vi "file paths.vi"(6 "error in (no error)":errorcluster, 7 "file path control":T1) -> (1 "ini":T2, 2 "coaglog":refnum<k34>, 4 "error out":errorcluster, 5 "datalog":refnum<k34>)   [LabVIEW 2019]
uses:
  <vilib>/Utility/config.llb/Config Data RefNum.ctl
  file paths.ctl
  <vilib>/Utility/config.llb/NI_LVConfig.lvlib
panel:
  out "appended path":path
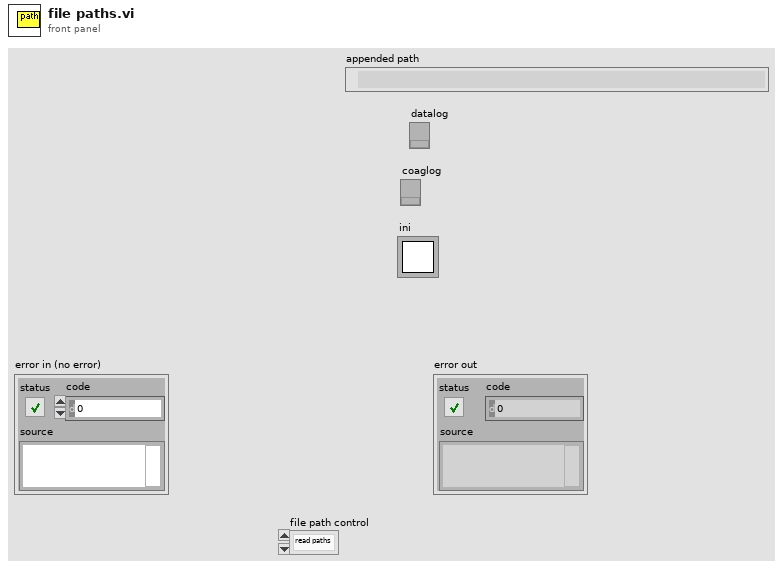
[diagram p1: front panel]
types:
  T1 = typedef "file paths.ctl" = enum16{"read paths", "close"}
  T2 = typedef "NI_LVConfig.lvlib/Config Data RefNum.ctl" = refnum<k1>
  T3 = enum16{"open", "open or create", "create or replace", "create", "open (read-only)"}
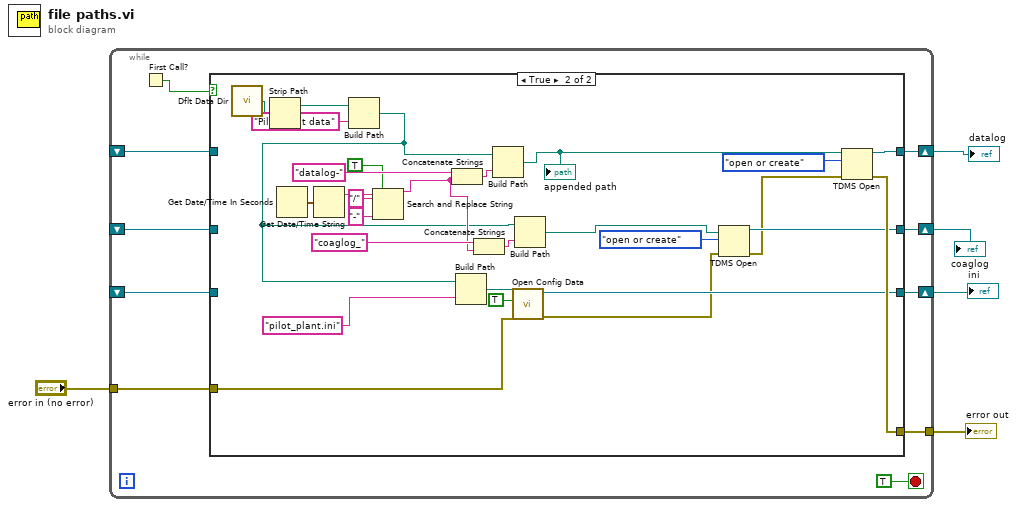
[diagram p0: block diagram]
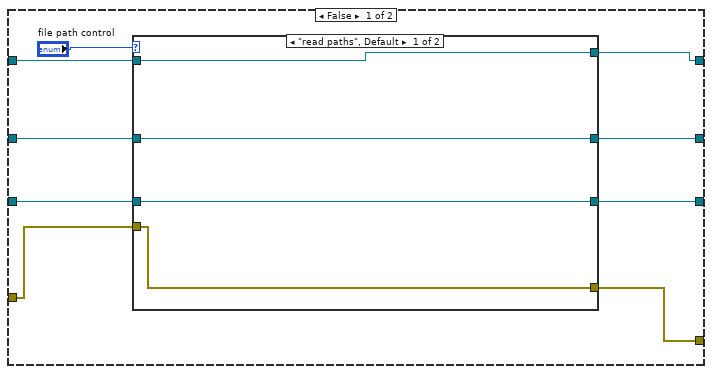
[diagram p2: hidden frame]
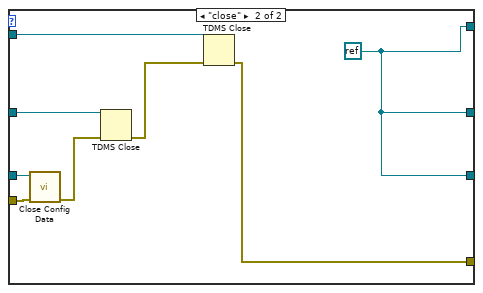
[diagram p3: hidden frame]
diagram:
  n1 = while {
    shift-right: [w15] -> w5
    shift-left: _ -> [w14]
    tunnel: "error in (no error)" -> [w13]
    tunnel: [w12] -> w3
    shift-right: [w10] -> w2
    shift-left: _ -> [w7]
    shift-right: [w9] -> w1
    shift-left: _ -> [w8]
    stop <- TRUE stop-if-true
    n2 = First Call?() -> (First Call?: T/F=w6:bool)
    n3 = case shown="True" w6 {
      tunnel: [w23 w63] -> w15
      tunnel: w14 -> [w22 _]
      tunnel: w13 -> [w17 w50]
      tunnel: [w16 w62] -> w12
      tunnel: [w19 w55] -> w10
      tunnel: [w21 w51] -> w9
      tunnel: w8 -> [w20 _]
      tunnel: w7 -> [w18 _]
      frame False {
        n4 = case shown="\"read paths\", Default" "file path control" {
          tunnel: [w28 w33] -> w23
          tunnel: w22 -> [w28 w36]
          tunnel: [w27 w33] -> w21
          tunnel: w20 -> [w27 w35]
          tunnel: [w26 w33] -> w19
          tunnel: w18 -> [w26 w34]
          tunnel: w17 -> [w25 w32]
          tunnel: [w25 w29] -> w16
          frame "read paths", Default {
          }
          frame "close" {
            w33 = refnum<k0> refnum
            n5 = call <vilib>:"Close Config Data.vi"("error in (no error)"=w32, "refnum"=w34) -> ("error out"=w31:errorcluster)  [unwired: 8 in, 1 out]
            n6 = TDMS Close(8:w31, 11:w35) -> (0:w30:errorcluster)  [unwired: 1 out]
            n7 = TDMS Close(8:w30, 11:w36) -> (0:w29:errorcluster)  [unwired: 1 out]
          }
        }
      }
      frame True {
        n8 = call <vilib>:"Dflt Data Dir.vi"() -> ("App:Default Data Directory"=w40:path)
        n9 = Strip Path(path=w40) -> (stripped path=w39:path)  [unwired: 1 out]
        n10 = Get Date/Time In Seconds() -> (seconds since 1Jan1904=w61:timestamp)
        n11 = Get Date/Time String(seconds (now)=w61) -> (date string=w46:string)  [unwired: 2 in, 1 out]
        n12 = Build Path(base path=w39, name or relative path="Pilot Plant data") -> (appended path=w37:path)
        n13 = Search and Replace String(replace all?=TRUE ("replace all? (F)"), input string=w46, search string="/", replace string="-" ("replace string (\"\")")) -> (result string=w43:string)  [unwired: 4 in, 3 out]
        n14 = Concatenate Strings("datalog-" ("string"), w43) -> (w59:string)
        n15 = Build Path(base path=w37, name or relative path="pilot_plant.ini") -> (appended path=w56:path)
        n16 = Concatenate Strings("coaglog_" ("string"), w43) -> (w53:string)
        n17 = Build Path(base path=w37, name or relative path=w59) -> (appended path=w58:path)
        "appended path" <- w58
        n18 = call <vilib>:"Open Config Data.vi"("error in (no error)"=w50, "create file if necessary (T)"=TRUE, "configuration file path"=w56) -> ("error out"=w49:errorcluster, "refnum"=w55:T2)  [unwired: 6 in, 1 out]
        n19 = Build Path(base path=w37, name or relative path=w53) -> (appended path=w52:path)
        n20 = TDMS Open(8:w49, 10:T3."open or create" ("operation (0:open)"), 11:w52) -> (0:w48:errorcluster, 3:w51:refnum<k34>)  [unwired: 4 in]
        n21 = TDMS Open(8:w48, 10:T3."open or create" ("operation (0:open)"), 11:w58) -> (0:w62:errorcluster, 3:w63:refnum<k34>)  [unwired: 4 in]
      }
    }
  }
  "datalog" <- w5
  "error out" <- w3
  "ini" <- w2
  "coaglog" <- w1
